vi "UI1.vi"(9 "Cluster":T1={"signal type"=enum."Sine Wave", "frequency"=10.0, "amplitude"=1.0, "signal out"={"t0"=timestamp(0 s since 1904-01-01), "dt"=1.0, "Y"=[]}, "WavefromRefnum"=refnum}) -> ()   [LabVIEW 2011]
panel:
  in  "signal type":T2(ring)
  out "Waveform Graph":waveform(dbl)(graph)
  in  "Amp":dbl=1.0
  in  "Freq":dbl=10.1
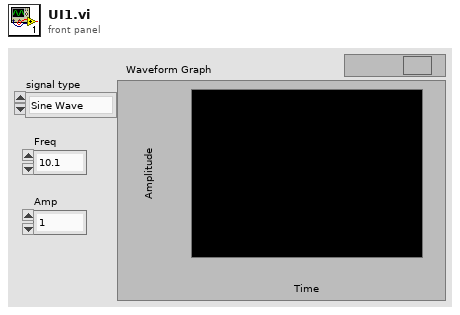
[diagram p1: front panel]
types:
  T1 = cluster{"signal type":enum16{"Sine Wave", "Triangle Wave", "Square Wave", "Sawtooth Wave"}, "frequency":dbl, "amplitude":dbl, "signal out":waveform(dbl), "WavefromRefnum":refnum<vi>}
  T2 = enum16{"Sine Wave", "Triangle Wave", "Square Wave", "Sawtooth Wave"}
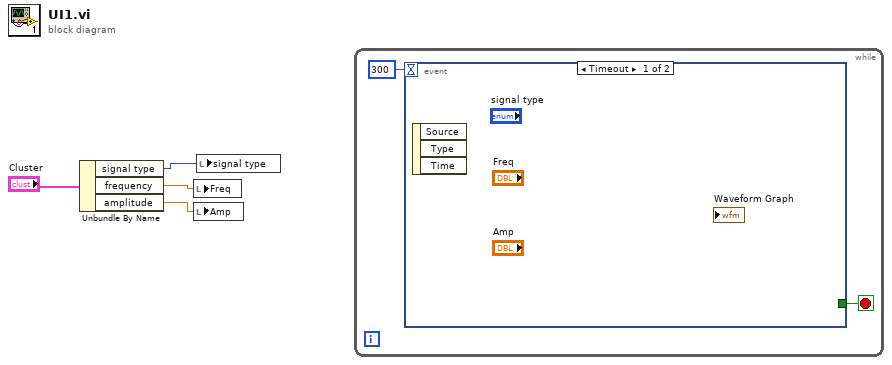
[diagram p0: block diagram]
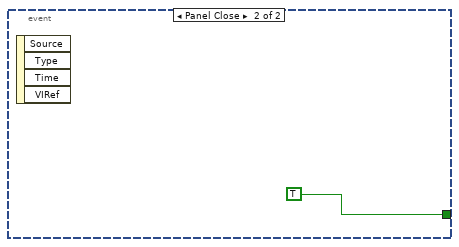
[diagram p2: hidden frame]
diagram:
  n1 = Unbundle By Name("Cluster") -> ("signal type"=w3:T2, "frequency"=w2:dbl, "amplitude"=w1:dbl)
  n2 = local write "Freq"(w2) -> ()
  n3 = local write "Amp"(w1) -> ()
  n4 = local write "signal type"(w3) -> ()
  n5 = while {
    stop <- w5 stop-if-true
    n6 = event shown="[0] Timeout" {
      selector: _ -> [_ _]
      dyn-events: _ -> [_ _]
      timeout: 300 -> [_ _]
      tunnel: [_ TRUE ("Discard?")] -> w5
      event Timeout {
        n7 = event-data() -> ()  [unwired: 1 in, 3 out]
      }
      event Panel Close {
        n8 = event-data() -> ()  [unwired: 1 in, 4 out]
      }
    }
  }
